vi "List Directory.vi"(8 "error in":errorcluster, 10 "Path":string, 11 "Session in":refnum<class "Session.lvclass">) -> (0 "error out":errorcluster, 1 "Items Count":i32, 2 "Items":T1[](array[typedef]))   [LabVIEW 2015, in "WinSCP.lvlib" / "Session.lvclass"]
uses:
  Session.lvclass
  ListDirectory-Item.ctl
  Session.lvclass/Session.ctl
  C:/Program Files (x86)/WinSCP/WinSCPnet.dll
  Program Files (x86)/WinSCP/WinSCPnet.dll
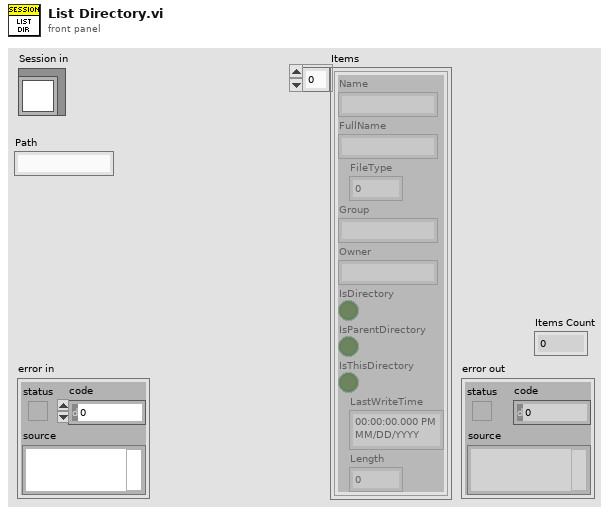
[diagram p1: front panel]
types:
  T1 = typedef "WinSCP.lvlib/Session.lvclass/ListDirectory-Item.ctl" = cluster{"Name":string, "FullName":string, "FileType":u16, "Group":string, "Owner":string, "IsDirectory":bool, "IsParentDirectory":bool, "IsThisDirectory":bool, "LastWriteTime":timestamp, "Length":i64}
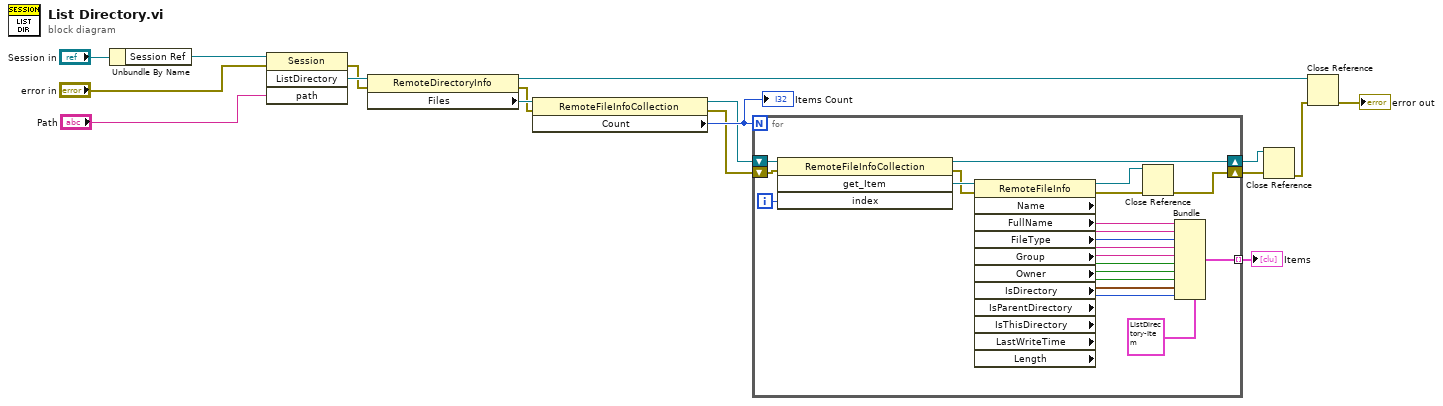
[diagram p0: block diagram]
diagram:
  n1 = Unbundle By Name("Session in") -> ("Session Ref"=w4:refnum<k24>)
  n2 = invoke class="Session" method="ListDirectory"(reference=w4, error in="error in", "path"="Path") -> (error out=w6:errorcluster, "ListDirectory"=w15:refnum<k24>)  [unwired: 1 in, 2 out]
  n3 = property class="RemoteDirectoryInfo"(reference=w15, error in=w6) -> (reference out=w7:refnum<k24>, error out=w5:errorcluster, "Files"=w14:refnum<k24>)
  n4 = property class="RemoteFileInfoCollection"(reference=w14, error in=w5) -> (reference out=w12:refnum<k24>, error out=w11:errorcluster, "Count"=w13:i32)
  "Items Count" <- w13
  n5 = for {
    N: w13 -> [_]
    shift-right: [w38] -> w9
    shift-left: w12 -> [w37]
    tunnel: [w25] -> w1 mode=indexing
    shift-right: [w20] -> w10
    shift-left: w11 -> [w22]
    i -> [w19]
    n6 = invoke class="RemoteFileInfoCollection" method="get_Item"(reference=w37, error in=w22, "index"=w19) -> (reference out=w38:refnum<k24>, error out=w21:errorcluster, "get_Item"=w36:refnum<k24>)  [unwired: 1 in, 1 out]
    n7 = property class="RemoteFileInfo"(reference=w36, error in=w21) -> (reference out=w24:refnum<k24>, error out=w23:errorcluster, "Name"=w35:string, "FullName"=w34:string, "FileType"=w33:u16, "Group"=w32:string, "Owner"=w31:string, "IsDirectory"=w30:bool, "IsParentDirectory"=w29:bool, "IsThisDirectory"=w28:bool, "LastWriteTime"=w27:timestamp, "Length"=w26:i64)
    n8 = Close Reference(reference=w24, error in (no error)=w23) -> (error out=w20:errorcluster)
    n9 = Bundle(cluster=T1 {"Name"="", "FullName"="", "FileType"=0, "Group"="", "Owner"="", "IsDirectory"=FALSE, "IsParentDirectory"=FALSE, "IsThisDirectory"=FALSE, "LastWriteTime"=timestamp(0 s since 1904-01-01), "Length"=0} ("Items"), "Name"=w35, "FullName"=w34, "FileType"=w33, "Group"=w32, "Owner"=w31, "IsDirectory"=w30, "IsParentDirectory"=w29, "IsThisDirectory"=w28, "LastWriteTime"=w27, "Length"=w26) -> (w25:T1)
  }
  "Items" <- w1
  n10 = Close Reference(reference=w9, error in (no error)=w10) -> (error out=w8:errorcluster)
  n11 = Close Reference(reference=w7, error in (no error)=w8) -> (error out=→"error out":errorcluster)
